vi "Open Altimeter Sensor.vi"(6 "I2C Slave Address":u8=236 format="%.0x", 7 "I2C Channel":u8, 8 "Error In":errorcluster, 11 "LINX Ref":T1) -> (0 "Error Out":errorcluster, 3 "LINX Resource":T1)   [LabVIEW 2014]
doc: "Open the I2C master and initialize the MMA8452 accelerometer.\n\nIf the LINX device has more than one I2C master the logical first I2C master is channel 0, the next is channel 1, etc."
uses:
  <vilib>/MakerHub/LINX/Private/Type Defs/LINX Ref.ctl
  <vilib>/MakerHub/LINX/Private/Type Defs/Platform.ctl
  <vilib>/MakerHub/LINX/Private/Type Defs/Interface.ctl
  <vilib>/MakerHub/LINX/Private/Device/Type Defs/LINX Device Config.ctl
  <vilib>/MakerHub/LINX/Private/Device/Type Defs/TCP Config.ctl
  <vilib>/MakerHub/LINX/Private/Device/Type Defs/Channels.ctl
  <vilib>/MakerHub/LINX/Private/Local IO/LinxI2cWrite.vi
  <vilib>/MakerHub/LINX/Public/Utilities/Check Channel.vi
  <vilib>/MakerHub/LINX/Private/Utilties/Generate Error.vi
  <vilib>/MakerHub/LINX/LMH-LINX.lvlib
  <vilib>/MakerHub/LINX/Private/Device/Device.lvlib
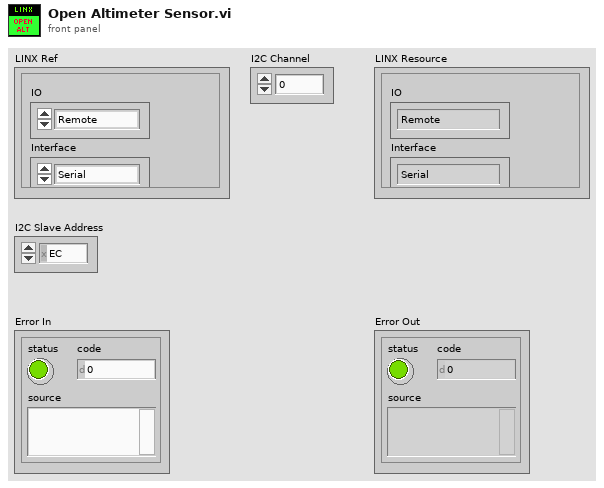
[diagram p1: front panel]
types:
  T1 = typedef "LMH-LINX.lvlib/LINX Ref.ctl" = cluster{"IO":T2, "Interface":T3, "LINX Device Config":T4}
  T2 = typedef "LMH-LINX.lvlib/Platform.ctl" = enum16{"Remote", "Local"}
  T3 = typedef "LMH-LINX.lvlib/Interface.ctl" = enum16{"Serial", "TCP"}
  T4 = typedef "LMH-LINX.lvlib/Device.lvlib/LINX Device Config.ctl" = cluster{"Interface":T3, "COM Port":refnum<visa-resource-name>, "TCP Configuration":T5, "Device Family":u8, "Device ID":u8, "Device Name":string, "TCP Ref":refnum<k5>, "Channels":T6}
  T5 = typedef "LMH-LINX.lvlib/Device.lvlib/TCP Config.ctl" = cluster{"IP Address":string, "Port":u16}
  T6 = typedef "LMH-LINX.lvlib/Channels.ctl" = cluster{"DI":u8[], "DO":u8[], "AI":u8[], "AO":u8[], "PWM":u8[], "QE":u8[], "UART":u8[], "I2C 2":u8[], "SPI":u8[], "CAN":u8[], "Servo":u8[], "AI Ref (V)":dbl, "AI Resolution (Bits)":u8, "AO Ref (V)":dbl, "AO Resolution (Bits)":u8}
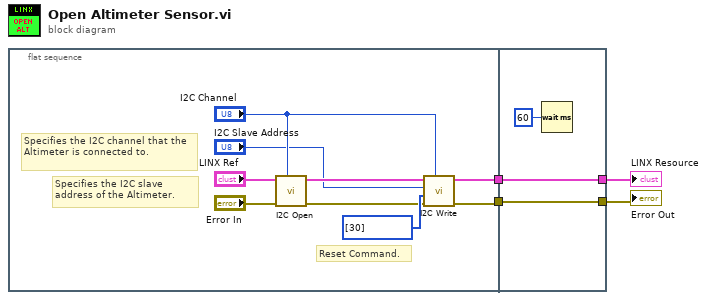
[diagram p0: block diagram]
diagram:
  n1 = flat-sequence {
    tunnel: [w6] -> w4
    tunnel: [w5] -> w2
    tunnel: w4 -> [w15]
    tunnel: [w15] -> w3
    tunnel: w2 -> [w14]
    tunnel: [w14] -> w1
    frame #0 {
      # "Specifies the I2C slave address of the Altimeter."
      # "Specifies the I2C channel that the Altimeter is connected to."
      # "Reset Command."
      n2 = call <vilib>:"I2C Open.vi"("I2C Channel (0)"="I2C Channel", "Error In"="Error In", "LINX Resource"="LINX Ref") -> ("Error Out"=w12:errorcluster, "LINX Resource"=w11:T1)  [unwired: 7 in]
      n3 = call <vilib>:"I2C Write.vi"("I2C Channel"="I2C Channel", "Error In"=w12, "Data"=u8[] [30], "I2C Slave Address (0)"="I2C Slave Address", "LINX Resource"=w11) -> ("Error Out"=w6:errorcluster, "LINX Resource"=w5:T1)  [unwired: 5 in]
    }
    frame #1 {
      n4 = Wait (ms)(milliseconds to wait=u32 60) -> ()  [unwired: 1 out]
    }
  }
  "LINX Resource" <- w1
  "Error Out" <- w3
